vi "ResMgr-ObtainBKThreadQ.vi"(8 "error in (no error)":errorcluster) -> (0 "error out":errorcluster, 3 "ObtainBKThreadQ":refnum<queue>)   [LabVIEW 2017, in "Communicable State Machine.lvlib"]
uses:
  Communicable State Machine.lvlib
  ResMgr-BackgroundThread.vi
  _Shared/CSM Shared.lvlib
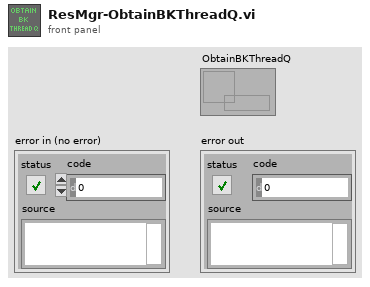
[diagram p1: front panel]
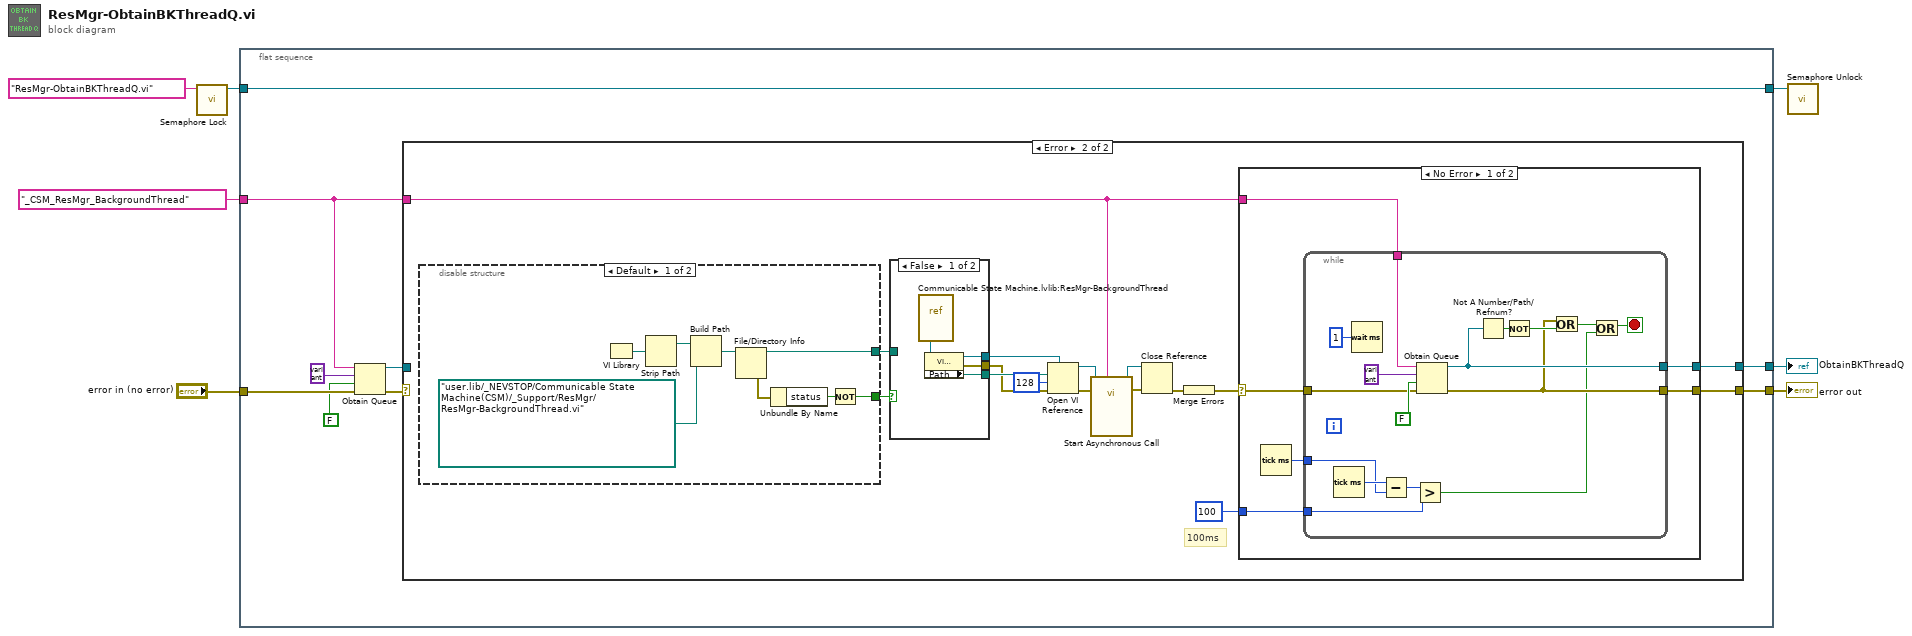
[diagram p0: block diagram]
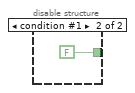
[diagram p4: hidden frame]
diagram:
  n1 = call "Semaphore Lock.vi"("name"="ResMgr-ObtainBKThreadQ.vi" ("name (unnamed)")) -> ("semaphore"=w2:refnum<queue>)  [unwired: 10 in]
  n2 = flat-sequence {
    tunnel: "error in (no error)" -> [w16]
    tunnel: "_CSM_ResMgr_BackgroundThread" ("name (unnamed)") -> [w15]
    tunnel: [w14] -> w5
    tunnel: [w13] -> w4
    tunnel: [w9] -> w3
    tunnel: w2 -> [w9]
    frame #0 {
      n3 = Obtain Queue(name (unnamed)=w15, element data type=variant, create if not found? (T)=FALSE, error in (no error)=w16) -> (queue out=w12:refnum<queue>, error out=w10:errorcluster)  [unwired: 1 in, 1 out]
      n4 = case shown="Error" w10 {
        selector: w10 -> [w17 _]
        tunnel: w12 -> [w18 _]
        tunnel: [w17 w25] -> w14
        tunnel: [w18 w23] -> w13
        tunnel: w15 -> [_ w22]
        frame No Error {
        }
        frame Error {
          # "100ms"
          n5 = disable-structure shown="Default" {
            disable-tunnel: [w42 FALSE ("file or folder exists?")] -> w20
            disable-tunnel: [w40 _] -> w19
            frame condition #0 (active) {
              n6 = VI Library() -> (path=w46:path)
              n7 = Strip Path(path=w46) -> (stripped path=w45:path)  [unwired: 1 out]
              n8 = Build Path(base path=w45, name or relative path=path "user.lib/_NEVSTOP/Communicable State Machine(CSM)/_Support/ResMgr/ResMgr-BackgroundThread.vi" ("<LabVIEW>")) -> (appended path=w41:path)
              n9 = File/Directory Info(path=w41) -> (path out=w40:path, error out=w44:errorcluster)  [unwired: 1 in, 5 out]
              n10 = Unbundle By Name(w44) -> ("status"=w43:bool)
              n11 = Not(x=w43) -> (.not. x?=w42:bool)
            }
            frame condition #1 {
            }
          }
          n12 = case shown="False" w20 {
            tunnel: [w37 w39] -> w33
            tunnel: [w36 _] -> w32
            tunnel: [w35 _] -> w30
            tunnel: w19 -> [_ w39]
            frame False {
              n13 = vi-ref "Communicable State Machine.lvlib:ResMgr-BackgroundThread.vi"() -> (w38:refnum<vi>)
              n14 = property class="VI (strict)"(reference=w38) -> (reference out=w35:refnum<vi>, error out=w36:errorcluster, "Path"=w37:path)  [unwired: 1 in]
            }
            frame True {
            }
          }
          n15 = Open VI Reference(type specifier VI Refnum (for type only)=w30, vi path=w33, options=128, error in (no error)=w32) -> (vi reference=w31:refnum<vi>, error out=w34:errorcluster)  [unwired: 2 in]
          n16 = call-by-ref "Start Asynchronous Call"(reference=w31, error in=w34, "name (unnamed)"=w22) -> (reference out=w28:refnum<vi>, error out=w29:errorcluster)  [unwired: 11 in]
          n17 = Close Reference(reference=w28, error in (no error)=w29) -> (error out=w26:errorcluster)
          n18 = Merge Errors(w26) -> (w24:errorcluster)
          n19 = case shown="No Error" w24 {
            selector: w24 -> [w53 w71]
            tunnel: [w54 w71] -> w25
            tunnel: [w52 _] -> w23
            tunnel: w22 -> [w51 _]
            tunnel: u32 100 ("y") -> [w49 _]
            frame No Error {
              n20 = Tick Count (ms)() -> (millisecond timer value=w50:u32)
              n21 = while {
                tunnel: [w67] -> w52
                tunnel: w51 -> [w68]
                tunnel: w50 -> [w61]
                tunnel: w49 -> [w59]
                tunnel: w53 -> [w69]
                tunnel: [w64] -> w54
                stop <- w57 stop-if-true
                n22 = Tick Count (ms)() -> (millisecond timer value=w62:u32)
                n23 = Wait (ms)(milliseconds to wait=u32 1) -> ()  [unwired: 1 out]
                n24 = Subtract(x=w62, y=w61) -> (x-y=w60:u32)
                n25 = Greater?(x=w60, y=w59) -> (0:w56:bool)
                n26 = Obtain Queue(name (unnamed)=w68, element data type=variant, create if not found? (T)=FALSE, error in (no error)=w69) -> (queue out=w67:refnum<queue>, error out=w64:errorcluster)  [unwired: 1 in, 1 out]
                n27 = Not A Number/Path/Refnum?(number/path/refnum=w67) -> (NaN/Path/Refnum?=w66:bool)
                n28 = Not(x=w66) -> (.not. x?=w65:bool)
                n29 = Or(x=w64, y=w65) -> (x .or. y?=w58:bool)
                n30 = Or(x=w58, y=w56) -> (x .or. y?=w57:bool)
              }
            }
            frame Error {
            }
          }
        }
      }
    }
  }
  n31 = call "Semaphore Unlock.vi"("semaphore"=w3) -> ()  [unwired: 11 in]
  "error out" <- w5
  "ObtainBKThreadQ" <- w4
